vi "Comunicacion.vi"(1 "Input cluster":T1) -> (0 "error out":errorcluster)   [LabVIEW 2014]
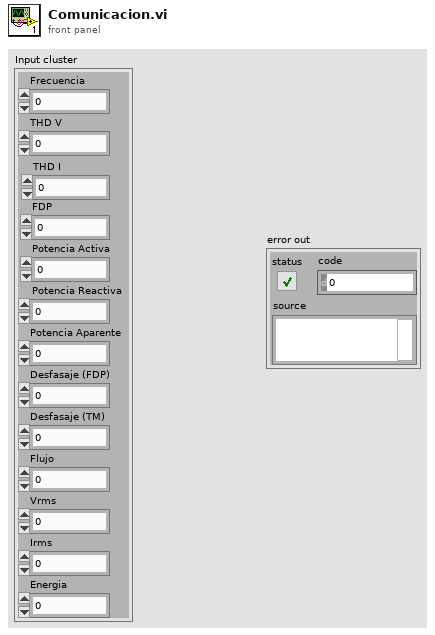
[diagram p1: front panel]
types:
  T1 = cluster{"Frecuencia":dbl, "THD V":dbl, "THD I":dbl, "FDP":dbl, "Potencia Activa":dbl, "Potencia Reactiva":dbl, "Potencia Aparente":dbl, "Desfasaje (FDP)":dbl, "Desfasaje (TM)":dbl, "Flujo":dbl, "Vrms":dbl, "Irms":dbl, "Energia":dbl}
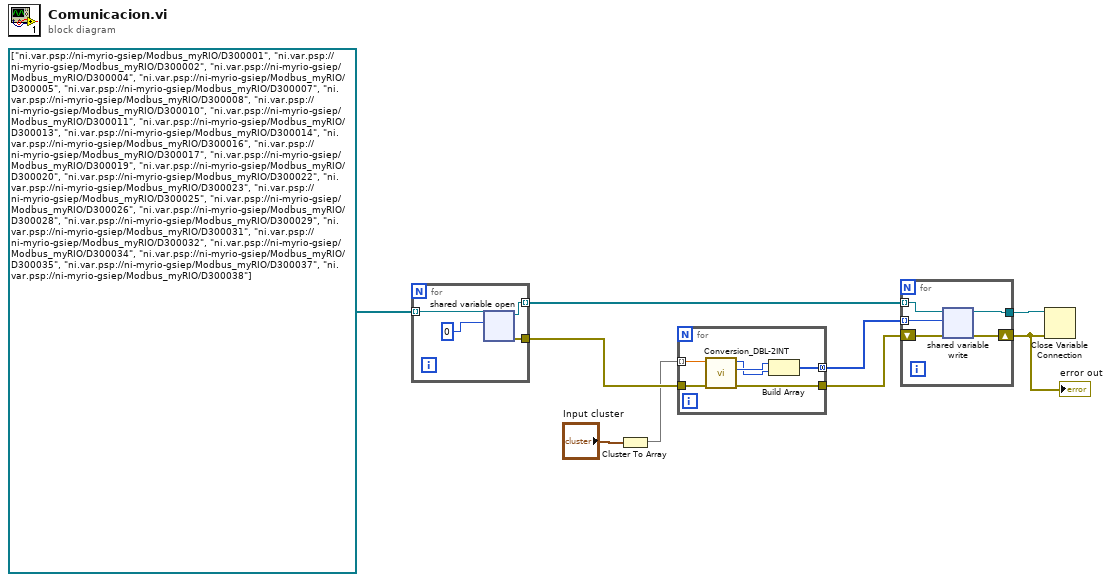
[diagram p0: block diagram]
diagram:
  n1 = for {
    tunnel: [w13] -> w1 mode=indexing
    tunnel: [w12] -> w5
    tunnel: refnum<k21>[] ["ni.var.psp://ni-myrio-gsiep/Modbus_myRIO/D300001", "ni.var.psp://ni-myrio-gsiep/Modbus_myRIO/D300002", "ni.var.psp://ni-myrio-gsiep/Modbus_myRIO/D300004", "ni.var.psp://ni-myrio-gsiep/Modbus_myRIO/D300005", "ni.var.psp://ni-myrio-gsiep/Modbus_myRIO/D300007", "ni.var.psp://ni-myrio-gsiep/Modbus_myRIO/D300008", "ni.var.psp://ni-myrio-gsiep/Modbus_myRIO/D300010", "ni.var.psp://ni-myrio-gsiep/Modbus_myRIO/D300011", "ni.var.psp://ni-myrio-gsiep/Modbus_myRIO/D300013", "ni.var.psp://ni-myrio-gsiep/Modbus_myRIO/D300014", "ni.var.psp://ni-myrio-gsiep/Modbus_myRIO/D300016", "ni.var.psp://ni-myrio-gsiep/Modbus_myRIO/D300017", "ni.var.psp://ni-myrio-gsiep/Modbus_myRIO/D300019", "ni.var.psp://ni-myrio-gsiep/Modbus_myRIO/D300020", "ni.var.psp://ni-myrio-gsiep/Modbus_myRIO/D300022", "ni.var.psp://ni-myrio-gsiep/Modbus_myRIO/D300023", "ni.var.psp://ni-myrio-gsiep/Modbus_myRIO/D300025", "ni.var.psp://ni-myrio-gsiep/Modbus_myRIO/D300026", "ni.var.psp://ni-myrio-gsiep/Modbus_myRIO/D300028", "ni.var.psp://ni-myrio-gsiep/Modbus_myRIO/D300029", "ni.var.psp://ni-myrio-gsiep/Modbus_myRIO/D300031", "ni.var.psp://ni-myrio-gsiep/Modbus_myRIO/D300032", "ni.var.psp://ni-myrio-gsiep/Modbus_myRIO/D300034", "ni.var.psp://ni-myrio-gsiep/Modbus_myRIO/D300035", "ni.var.psp://ni-myrio-gsiep/Modbus_myRIO/D300037", "ni.var.psp://ni-myrio-gsiep/Modbus_myRIO/D300038"] -> [w10] mode=indexing
    n2 = shared-variable-open(w10, u32 0) -> (w13:refnum<k21>, w12:errorcluster)  [unwired: 2 in]
  }
  n3 = Cluster To Array(cluster="Input cluster") -> (array=w3:dbl[])
  n4 = for {
    tunnel: w3 -> [w19] mode=indexing
    tunnel: [w18] -> w6 mode=concatenating
    tunnel: w5 -> [w15]
    tunnel: [w14] -> w4
    n5 = call "Conversion_DBL-2INT.vi"("error in"=w15, "Double"=w19) -> ("error out"=w14:errorcluster, "Integer LOW"=w17:u32, "Integer HIGH"=w16:u32)  [unwired: 2 in, 1 out]
    n6 = Build Array(w17, w16) -> (w18:u32[])
  }
  n7 = for {
    tunnel: [w23] -> w9
    tunnel: w6 -> [w21] mode=indexing
    shift-right: [w22] -> w8
    shift-left: w4 -> [w24]
    tunnel: w1 -> [w20] mode=indexing
    n8 = shared-variable-write(w20, w24, w21) -> (w23:refnum<k21>, w22:errorcluster)
  }
  "error out" <- w8
  n9 = Close Variable Connection(8:w8, 11:w9) -> ()  [unwired: 1 out]
